vi "Get Overload Protection Timeout.vi"(8 "error in (no error)":errorcluster, 11 "VISA resource name":refnum<visa-resource-name>) -> (0 "error out":errorcluster, 2 "Timeout Value":dbl format="%.4f", 3 "VISA resource name out":refnum<visa-resource-name>)   [LabVIEW 2011, in "Fluke 5XXX Series Multicalibrators.lvlib"]
doc: "This VI returns the programmed OPERATE time limit for the OVERLD mode signal.\n\nNote:\n\nThis VI is available only for instrument models 5500A and 5520A with oscilloscope option SC600 (SC1100)."
uses:
  Fluke 5XXX Series Multicalibrators.lvlib
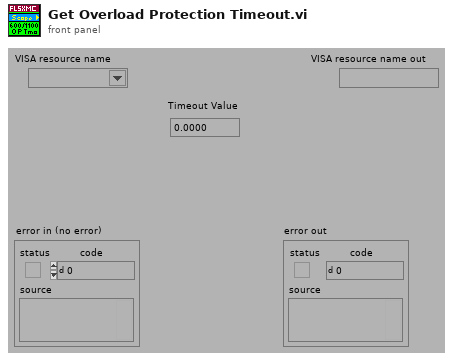
[diagram p1: front panel]
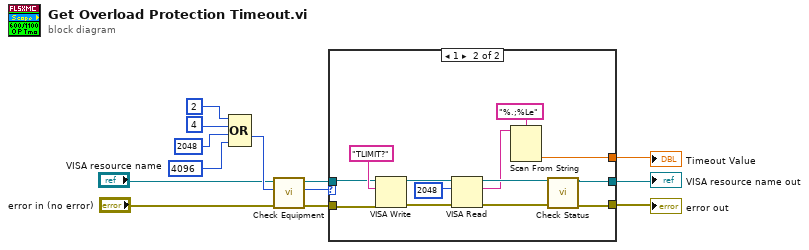
[diagram p0: block diagram]
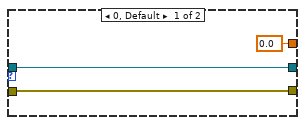
[diagram p2: hidden frame]
diagram:
  n1 = Compound Arithmetic op=OR(2 ("Numeric"), 4 ("Numeric"), 2048 ("Numeric"), 4096 ("Numeric")) -> (w7:i32)
  n2 = call "Check Equipment.vi"("error in (no error)"="error in (no error)", "Bit Mask"=w7, "VISA resource name"="VISA resource name") -> ("error out"=w10:errorcluster, "Present?"=w9:u32, "VISA resource name out"=w8:refnum<visa-resource-name>)  [unwired: 6 in]
  n3 = case shown="1" w9 {
    tunnel: [w15 w19] -> w2
    tunnel: w10 -> [w16 w21]
    tunnel: w8 -> [w15 w18]
    tunnel: [w16 w20] -> w3
    tunnel: [0.0 w17] -> w1
    frame 0, Default {
    }
    frame 1 {
      n4 = VISA Write(VISA resource name=w18, write buffer="TLIMIT?", error in (no error)=w21) -> (VISA resource name out=w27:refnum<visa-resource-name>, error out=w26:errorcluster)  [unwired: 1 out]
      n5 = VISA Read(VISA resource name=w27, byte count=u32 2048 ("byte count (0)"), error in (no error)=w26) -> (VISA resource name out=w24:refnum<visa-resource-name>, read buffer=w23:string, error out=w25:errorcluster)  [unwired: 1 out]
      n6 = Scan From String(format string="%.;%Le", input string=w23) -> (output 1=w17:dbl)  [unwired: 3 in, 3 out]
      n7 = call "Check Status.vi"("VISA resource name"=w24, "error in (no error)"=w25) -> ("VISA resource name out"=w19:refnum<visa-resource-name>, "error out"=w20:errorcluster)  [unwired: 12 in]
    }
  }
  "Timeout Value" <- w1
  "VISA resource name out" <- w2
  "error out" <- w3
